vi "DuraFET_Temp_CalibCalc.vi"(11 "Voltage from Thermistor":dbl) -> (1 "Resistance (Ohm)":dbl, 2 "Temperature (C)":dbl)   [LabVIEW 2018]
panel:
  # "INPUTS"
  # "OUTPUTS"
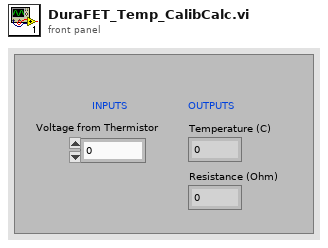
[diagram p1: front panel]
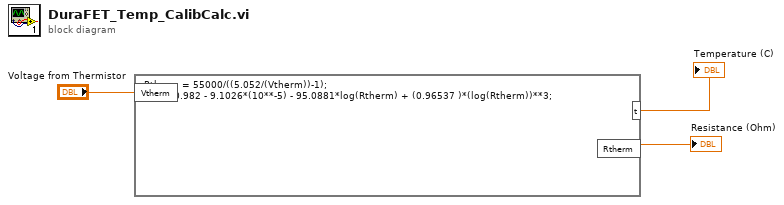
[diagram p0: block diagram]
diagram:
  n1 = formula code="Rtherm = 55000/((5.052/(Vtherm))-1);\nt = 340.982 - 9.1026*(10**-5) - 95.0881*log(Rtherm) + (0.96537 )*(log(Rtherm))**3;"("Vtherm"="Voltage from Thermistor") -> ("t"=→"Temperature (C)":dbl, "Rtherm"=→"Resistance (Ohm)":dbl)
